vi "SampleAvg.Accumulator.vi"(7 "Data":i32[](array[numeric])=[0, 0, 0, 0], 8 "Input Valid":bool, 9 "New Record":bool, 10 "NewCount?":bool, 11 "Count":i16) -> (1 "Acc Valid":bool, 2 "Accumulator":i32[](array[numeric]), 3 "End Count":i16)   [LabVIEW 2014]
doc: "<b> Latency = 3 Ticks </b>"
uses:
  <vilib>/rvi/FXPMathLib/basic elements/FxpIntAccumulator/subVIs/nifxpmath_IntAccumulator_SimConfig.ctl
  <vilib>/rvi/FXPMathLib/basic elements/FxpIntAccumulator/simVIs/DllFxpIntAccumulator_sub.vi
  <vilib>/rvi/FXPMathLib/basic elements/FxpIntAccumulator/XNode/nifxpmath_IntAccumulator.xnode
panel:
  # "Copyright 2014 Vidrio Technologies\nScanImage 5 software is licensed under the Apache License, Version 2.0 (the \"License\"); you may not use any files contained\nwithin the ScanImage 5 release except in compliance with the License. You may obtain a copy of the License at\n http://www.apache.org/licenses/LICENSE-2.0\nUnless required by applicable law or agreed to in writing, software distributed under the License is distributed on an\n\"AS IS\" BASIS, WITHOUT WARRANTIES OR CONDITIONS OF ANY KIND, either express or implied. See the License for the\n specific language governing permissions and limitations under the License."
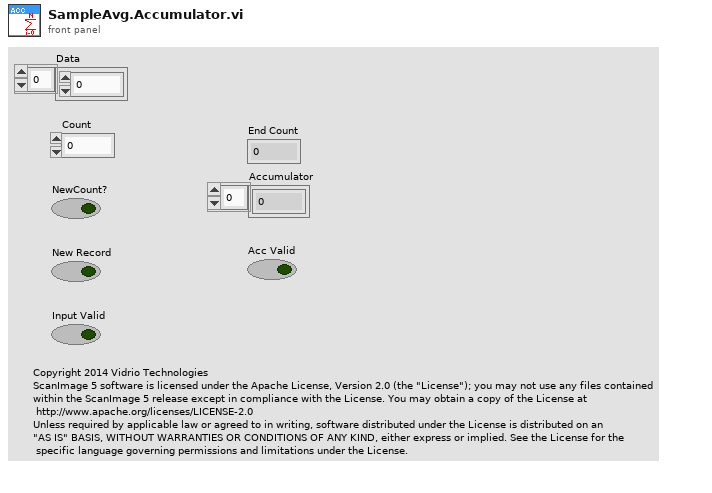
[diagram p1: front panel]
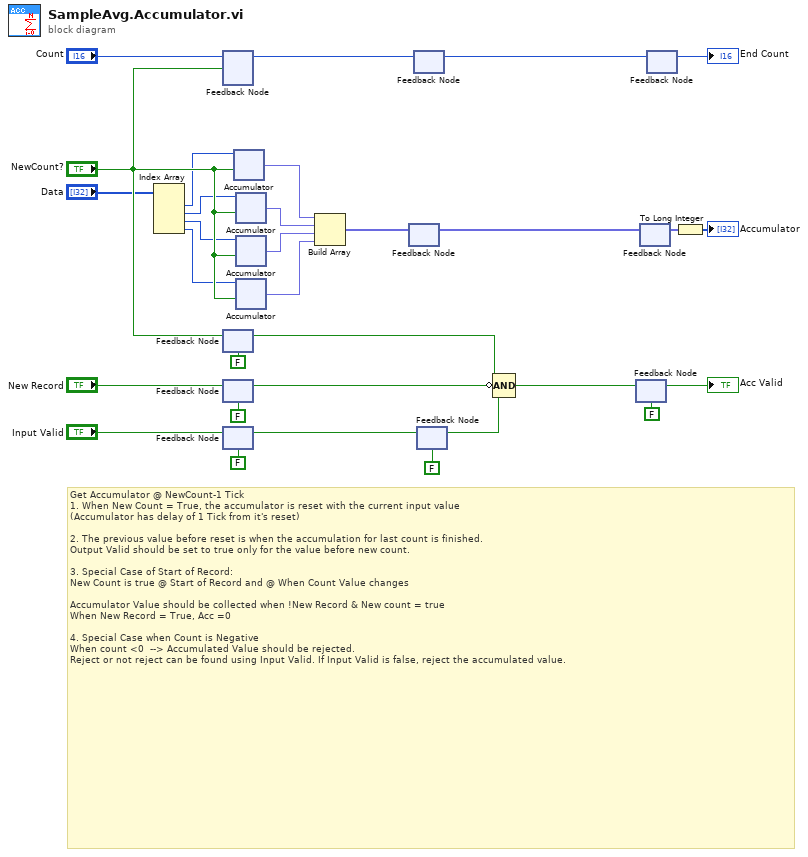
[diagram p0: block diagram]
diagram:
  # "Get Accumulator @ NewCount-1 Tick\n1. When New Count = True, the accumulator is reset with the current input value\n(Accumulator has delay of 1 Tick from it's reset)\n\n2. The previous value before reset is when the accumulation for last count is finished.\nOutput Valid should be set to true only for the value before new count.\n\n3. Special Case of Start of Record:\nNew Count is true @ Start of Record and @ When Count Value changes\n\nAccumulator Value should be collected when !New Record & New count = true\nWhen New Record = True, Acc =0\n\n4. Special Case when Count is Negative\nWhen count <0  --> Accumulated Value should be rejected.\nReject or not reject can be found using Input Valid. If Input Valid is false, reject the accumulated value."
  n1 = Index Array(array="Data") -> (element #1=w9:i32, element #2=w8:i32, element #3=w7:i32, element #4=w6:i32)  [unwired: 4 in]
  n2 = feedback #1() -> (w20:i16)  [unwired: 1 in]
  n3 = feedback-in #1("Count", "NewCount?") -> ()
  n4 = feedback #2(FALSE ("NewCount?")) -> (w29:bool)
  n5 = feedback-in #2("NewCount?") -> ()
  n6 = feedback #3(FALSE ("NewCount?")) -> (w28:bool)
  n7 = feedback-in #3("New Record") -> ()
  n8 = feedback #4(FALSE ("NewCount?")) -> (w24:bool)
  n9 = feedback-in #4("Input Valid") -> ()
  n10 = xnode "Accumulator"("x"=w9, "load (F)"="NewCount?") -> ("s"=w5:fxp<+/-,32,32>)  [unwired: 3 in, 1 out]
  n11 = xnode "Accumulator"("x"=w8, "load (F)"="NewCount?") -> ("s"=w4:fxp<+/-,32,32>)  [unwired: 3 in, 1 out]
  n12 = xnode "Accumulator"("x"=w7, "load (F)"="NewCount?") -> ("s"=w3:fxp<+/-,32,32>)  [unwired: 3 in, 1 out]
  n13 = xnode "Accumulator"("x"=w6, "load (F)"="NewCount?") -> ("s"=w2:fxp<+/-,32,32>)  [unwired: 3 in, 1 out]
  n14 = Build Array(w5, w4, w3, w2) -> (w1:fxp<+/-,32,32>[])
  n15 = feedback-in #5(w1) -> ()
  n16 = feedback #5() -> (w19:fxp<+/-,32,32>[])  [unwired: 1 in]
  n17 = feedback #6() -> (w18:i16)  [unwired: 1 in]
  n18 = feedback-in #6(w20) -> ()
  n19 = feedback #7(FALSE ("NewCount?")) -> (w13:bool)
  n20 = feedback-in #7(w24) -> ()
  n21 = Compound Arithmetic op=AND(w29, invert w28, w13) -> (w27:bool)
  n22 = feedback-in #8(w27) -> ()
  n23 = feedback #8(FALSE) -> (→"Acc Valid":bool)
  n24 = feedback-in #9(w19) -> ()
  n25 = feedback #9() -> (w16:fxp<+/-,32,32>[])  [unwired: 1 in]
  n26 = feedback-in #10(w18) -> ()
  n27 = feedback #10() -> (→"End Count":i16)  [unwired: 1 in]
  n28 = To Long Integer(number=w16) -> (32bit integer=→"Accumulator":i32[])
